vi "peak -- draw -- fit related.vi"() -> ()   [LabVIEW 2010]
uses:
  circle corners.ctl
  lorentzian.ctl
  wavepacket.ctl
  complex region.ctl
panel:
  in  "complex region 2":T1
  in  "parameters: wavepacket  2":T2={"R"=0.5, "wave number"=22.0, "delta k"=7.0, "radii vector"=[], "radial section"=[], "wave vector"=22.0, "wavepacket is"=TRUE} {"delta k" format="%#_3f"; "wave number" format="%#_3f"; "R" format="%#_3f"}
  in  "lorentzian":T3={"Amplitude"=-1.0311345636926572, "omega(0)"=-1.0311345636926572, "Gamma"=-1.0311345636926572, "phase"=-1.0311345636926572, "Q"=-1.0311345636926572, "Norm  Ampl"=-1.0311345636926572, "z (inf)"=-1.0311345636926572+0.0i, "4corners"={"z (-pi/2)"=-1.0311345636926572+0.5736824521422934i, "z(inf)"=-0.5200164984937075+1.0975277942502903i, "z (pi/2)"=-1.0311345636926572+0.5736824521422934i, "z center"=-0.5136528600391839+0.580046090596817i, "z(0)"=-0.5200164984937075+1.0975277942502903i, "radius"=-1.0311345636926572}} {"z (inf)" format="%#9_9f"; "Q" format="%#9_9f"; "phase" format="%#9_9f"; "Gamma" format="%#9_9f"; "omega(0)" format="%#9_9f"}
  out "Plot: complex plane":cluster{dbl[], dbl[]}[](graph)=[{array[1389 elements], array[1389 elements]}, {[0.4353850246464146, 0.43182331903139287, 0.4211943724115363, 0.403665809624465, 0.379514066576387, 0.3491200306827224, 0.3129630340460312, 0.27161329410241697, 0.22572292095192775, 0.176015633192727, 0.12327534444647162, 0.06833380057221139, 0.012057462537330959, -0.04466615818950484, -0.10094249622438536, -0.1558840400986455, -0.20862432884490087, -0.25833161660410175, -0.3042219897545908, -0.3455717296982051, -0.3817287263348962, -0.4121227622285608, -0.43627450527663886, -0.4538030680637101, -0.4644320146835667, -0.46799372029858843, -0.4644320146835667, -0.4538030680637101, -0.4362745052766388, -0.41212276222856076, -0.38172872633489613, -0.34557172969820504, -0.30422198975459075, -0.25833161660410153, -0.20862432884490062, -0.1558840400986455, -0.10094249622438527, -0.04466615818950476, 0.012057462537331146, 0.06833380057221167, 0.12327534444647154, 0.17601563319272698, 0.22572292095192786, 0.2716132941024171, 0.3129630340460314, 0.3491200306827225, 0.379514066576387, 0.403665809624465, 0.42119437241153634, 0.43182331903139287], [0.016304347826086918, 0.07291603744469696, 0.1286349268998374, 0.18258229601994944, 0.2339073625674127, 0.28180069958266507, 0.32550700053088333, 0.36433699093723537, 0.39767829865710114, 0.4250051113506065, 0.44588646885732824, 0.4599930596954671, 0.4671024145006366, 0.4671024145006366, 0.45999305969546705, 0.44588646885732824, 0.4250051113506065, 0.3976782986571011, 0.36433699093723537, 0.3255070005308833, 0.2818006995826651, 0.23390736256741268, 0.18258229601994933, 0.1286349268998374, 0.07291603744469691, 0.016304347826086772, -0.04030734179252315, -0.09602623124766366, -0.14997360036777574, -0.2012986669152389, -0.24919200393049135, -0.2928983048787095, -0.3317282952850616, -0.36506960300492736, -0.39239641569843275, -0.4132777732051544, -0.4273843640432933, -0.4344937188484628, -0.4344937188484628, -0.4273843640432932, -0.41327777320515446, -0.39239641569843264, -0.36506960300492725, -0.3317282952850614, -0.2928983048787093, -0.249192003930491, -0.20129866691523887, -0.14997360036777554, -0.09602623124766342, -0.040307341792522926]}, {[-0.02920754195733423, -0.0279172225442095, -0.02662690313108477, -0.025336583717960035, -0.024046264304835304, -0.022755944891710574, -0.021465625478585843, -0.020175306065461113, -0.01888498665233638, -0.017594667239211652, -0.016304347826086918, -0.015014028412962187, -0.013723708999837457, -0.012433389586712727, -0.011143070173587993, -0.009852750760463262, -0.008562431347338532, -0.007272111934213801, -0.005981792521089071, -0.004691473107964337], [-0.4352006873460732, -0.3900501838288572, -0.3448996803116412, -0.29974917679442514, -0.25459867327720914, -0.20944816975999314, -0.16429766624277709, -0.11914716272556108, -0.07399665920834508, -0.028846155691129083, 0.016304347826086918, 0.061454851343302974, 0.10660535486051903, 0.15175585837773498, 0.19690636189495103, 0.24205686541216698, 0.28720736892938303, 0.3323578724465991, 0.37750837596381503, 0.4226588794810311]}, {[-0.46780938299824704, -0.42265887948103104, -0.37750837596381503, -0.332357872446599, -0.287207368929383, -0.24205686541216698, -0.19690636189495092, -0.15175585837773492, -0.10660535486051892, -0.06145485134330292, -0.016304347826086918, 0.02884615569112914, 0.0739966592083452, 0.11914716272556114, 0.1642976662427772, 0.20944816975999314, 0.2545986732772092, 0.29974917679442525, 0.3448996803116412, 0.39005018382885726], [0.02920754195733423, 0.0279172225442095, 0.02662690313108477, 0.025336583717960035, 0.024046264304835304, 0.022755944891710574, 0.021465625478585843, 0.020175306065461113, 0.01888498665233638, 0.017594667239211652, 0.016304347826086918, 0.015014028412962187, 0.013723708999837457, 0.012433389586712727, 0.011143070173587993, 0.009852750760463262, 0.008562431347338532, 0.007272111934213801, 0.005981792521089071, 0.004691473107964337]}, {[0.01005665579823264, 0.007744432577840361, 0.005417179652517198, 0.003076351479586171, 0.0007234110004580747, -0.0016401712736591172, -0.00401291818078202, -0.006393346831329957, -0.008779969534882585, -0.011171294729938152, -0.013565827916090699, -0.015962072588044322, -0.018358531170880203, -0.02075370595599212, -0.023146100037105728, -0.025534218245796075, -0.027916568085919358, -0.030291660666374353, -0.032658011631610834, -0.03501414208930362], [0.10847338189925305, 0.10910353702052725, 0.10967569566929894, 0.11018950026503718, 0.11064462969659473, 0.11104079952289196, 0.11137776215068329, 0.11165530698929499, 0.11187326058223739, 0.1120314867156096, 0.11212988650322873, 0.11216839844843059, 0.11214699848250304, 0.11206569997972819, 0.11192455374902387, 0.1117236480021898, 0.11146310829877795, 0.11114309746762203, 0.11076381550507473, 0.11032549945001648]}, {[0.014540048997765252, 0.011834570421475052, 0.00911150593724143, 0.006372557371727504, 0.003619436478630049, 0.0008538638688893457, -0.0019224320646368132, -0.0047077162273623414, -0.007500247907350391, -0.010298281863201853, -0.013100069414774205, -0.015903859536049864, -0.018707899949470363, -0.021510438221052725, -0.024309722855603812, -0.027104004391347636, -0.029891536493282165, -0.0326705770445818, -0.03543938923536362, -0.038196242648137146], [0.12414918948458693, 0.12488651932597554, 0.125555988844679, 0.12615717964404025, 0.12668971599937934, 0.12715326509280894, 0.12754753722123485, 0.12787228597741096, 0.1281273084039356, 0.12831244512009365, 0.12842758042146385, 0.12847264235223071, 0.12844760275015438, 0.128352477264171, 0.1281873253446129, 0.12795225020605383, 0.1276473987628034, 0.12727296153709028, 0.1268291725399921, 0.1263163091251861]}]
  out "Plot: linear map":cluster{dbl[], dbl[]}[](graph)
  out "Plot: geometry":cluster{dbl, dbl}[](graph)
  out "Plot: phase around center":cluster{dbl[], dbl[]}[](graph)=[{array[1389 elements], array[1389 elements]}, {[3015.8552146531347, 3016.2383756063605, 3016.6215365595863], [1.7830935388456814, 3.353889865640578, 4.924686192435475]}, {array[1389 elements], array[1389 elements]}]
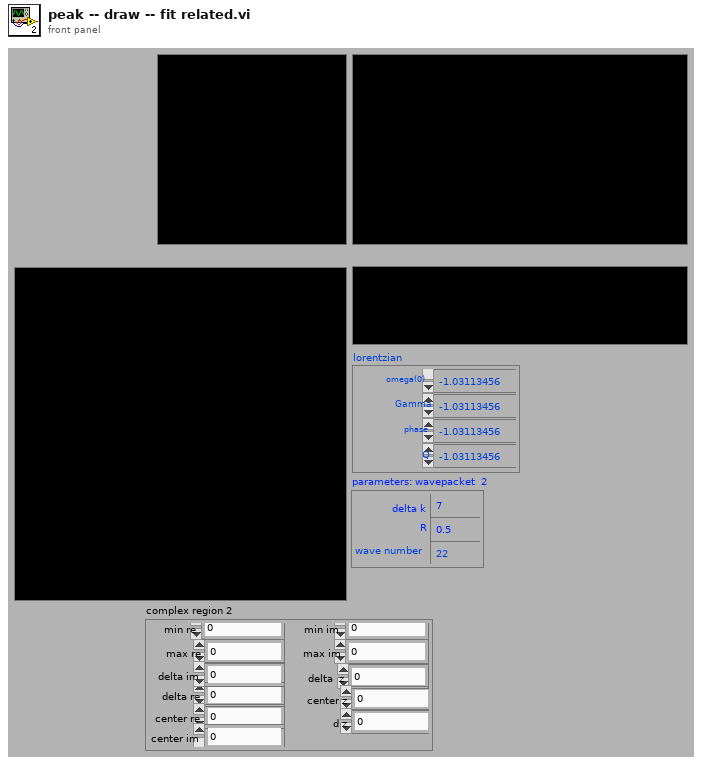
[diagram p1: front panel]
types:
  T1 = typedef "complex region.ctl" = cluster{"max re":dbl, "min re":dbl, "max im":dbl, "min im":dbl, "delta re":dbl, "delta im":dbl, "center re":dbl, "delta  z":cdb, "center im":dbl, "center z":cdb, "d im":dbl, "d re":dbl, "d z":cdb}
  T2 = typedef "wavepacket.ctl" = cluster{"R":dbl, "wave number":dbl, "delta k":dbl, "radii vector":dbl[], "radial section":cdb[], "wave vector":dbl, "wavepacket is":bool}
  T3 = typedef "lorentzian.ctl" = cluster{"Amplitude":dbl, "omega(0)":dbl, "Gamma":dbl, "phase":dbl, "Q":dbl, "Norm  Ampl":dbl, "z (inf)":cdb, "4corners":T4}
  T4 = typedef "circle corners.ctl" = cluster{"z (-pi/2)":cdb, "z(inf)":cdb, "z (pi/2)":cdb, "z center":cdb, "z(0)":cdb, "radius":dbl}
  T5 = typedef "single fit parameters.ctl" = cluster{"number of 2D grid points":i32, "# of points in pond":i32, "# of points in window":i32, "decimation threshold":i32, "normalization factor":dbl, "pond scale factor ":dbl, "normalized z":cdb[], "decimated z":cdb[], "decimated omega":dbl[], "omega in window":dbl[], "z in window":cdb[], "data center":cdb, "inverse":cdb[], "linear ":cdb[], "omega around":dbl[], "phase around center":dbl[], "fit for phase around senter ":dbl[], "three points":cluster{dbl[], dbl[]}, "max omega":dbl, "min omega":dbl}
  T6 = typedef "omega map parameters.ctl" = cluster{"map method":enum16{"simple", "less trivial", "around center", "geometry"}, "2:window factor":i32, "left":dbl, "right":dbl, "omega":dbl, "gamma":dbl, "theta0":dbl, "use points":enum16{"all in window", "decimated"}, "z(inf) method":enum16{"median", "method 2", "histogram"}}
  T7 = cluster{"omega in window":void, "phase around center":void}
  T8 = cluster{"omega in window":void, "f(X,a)":dbl[]}[]
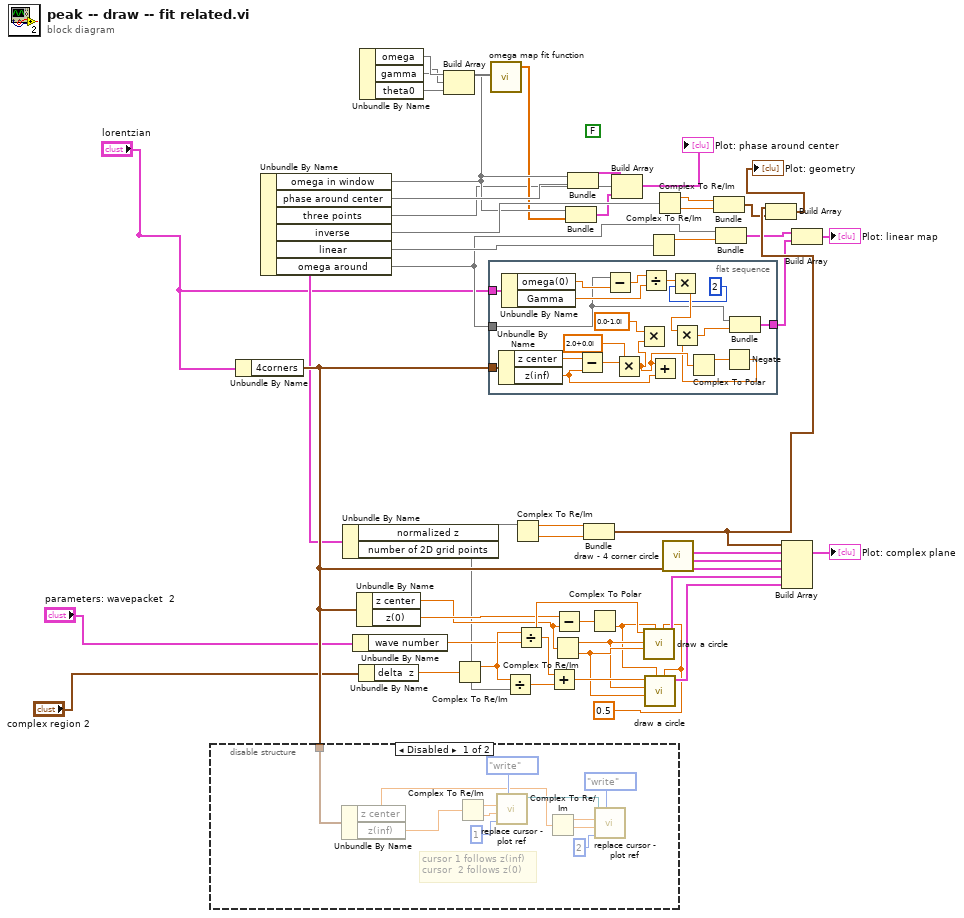
[diagram p0: block diagram]
diagram:
  w14 = 0.5
  (unwired) FALSE
  n1 = Unbundle By Name("lorentzian") -> ("4corners"=w50:T4)
  n2 = disable-structure shown="Disabled" {
    disable-tunnel: w50 -> [w65 _]
    frame Disabled {
      # "cursor 1 follows z(inf)\ncursor  2 follows z(0)"
      n3 = Unbundle By Name(w65) -> ("z center"=w53:cdb, "z(inf)"=w54:cdb)
      n4 = Complex To Re/Im(x + iy=w54) -> (x=w61:dbl, y=w60:dbl)
      n5 = call "replace cursor - plot ref.vi"("action"=enum16{"", "read", "write"}."write" ("Enum"), "cursor index"=1, "new  Y"=w60, "new X"=w61) -> ("Plot ref out"=w55:refnum<vi>, "Plot ref in"=w64:refnum<vi>)  [unwired: 4 in, 2 out]
      n6 = Complex To Re/Im(x + iy=w53) -> (x=w57:dbl, y=w56:dbl)
      n7 = call "replace cursor - plot ref.vi"("action"=enum16{"", "read", "write"}."write" ("Enum"), "cursor index"=2, "new  Y"=w56, "new X"=w57, "Plot ref in"=w55) -> ()  [unwired: 4 in, 3 out]
    }
    frame Enabled {
    }
  }
  n8 = Unbundle By Name() -> (w49:T5, "omega in window"=w30, "phase around center"=w37, "three points"=w28, "inverse"=w41, "linear"=w40, "omega around"=w39)
  n9 = Unbundle By Name(w49) -> ("normalized z"=w9, "number of 2D grid points"=w4)
  n10 = Unbundle By Name("parameters: wavepacket  2") -> ("wave number"=w10:dbl)
  n11 = Unbundle By Name(w50) -> ("z center"=w5:cdb, "z(0)"=w17:cdb)
  n12 = Unbundle By Name("complex region 2") -> ("delta  z"=w11:cdb)
  n13 = Unbundle By Name() -> (w51:T6, "omega"=w34, "gamma"=w33, "theta0"=w32)
  n14 = Build Array(w34, w33, w32) -> (w31:void[])
  n15 = Complex To Re/Im(x + iy=w11) -> (x=w12:dbl)  [unwired: 1 out]
  n16 = flat-sequence {
    tunnel: "lorentzian" -> [w84]
    tunnel: w50 -> [w83]
    tunnel: w39 -> [w72]
    tunnel: [w71] -> w38
    frame #0 {
      n17 = Unbundle By Name(w83) -> ("z center"=w82:cdb, "z(inf)"=w80:cdb)
      n18 = Unbundle By Name(w84) -> ("omega(0)"=w78:dbl, "Gamma"=w76:dbl)
      n19 = Subtract(x=w82, y=w80) -> (x-y=w81:cdb)
      n20 = Subtract(x=w72, y=w78) -> (x-y=w77:dbl)
      n21 = Multiply(x=w81, y=cdb 2.0+0.0i) -> (x*y=w68:cdb)
      n22 = Multiply(x=cdb 0.0-1.0i ("y"), y=w68) -> ()  [unwired: 1 out]
      n23 = Divide(x=w77, y=w76) -> (x/y=w75:dbl)
      n24 = Add(x=w68, y=w80) -> ()  [unwired: 1 out]
      n25 = Multiply(x=w75, y=2) -> (x*y=w73:dbl)
      n26 = Complex To Polar(r * e^(i*theta)=w68) -> (r=w67:dbl)  [unwired: 1 out]
      n27 = Negate(x=w67) -> (-x=w66:dbl)
      n28 = Multiply(x=w73, y=w66) -> (x*y=w69:dbl)
      n29 = Bundle("omega around"=w72, w69) -> (w71:cluster{"omega around":void, dbl})  [unwired: 1 in]
    }
  }
  n30 = call "omega map fit function.vi"("X"=w30, "a"=w31) -> ("f(X,a)"=w29:dbl[])  [unwired: 2 in, 2 out]
  n31 = Divide(x=w12, y=w4) -> (x/y=w13:dbl)
  n32 = Complex To Re/Im(x + iy=w9) -> (x=w26:dbl, y=w25:dbl)
  n33 = Divide(x=w12, y=w10) -> (x/y=w22:dbl)
  n34 = Add(x=w22, y=w13) -> (x+y=w21:dbl)
  n35 = Complex To Re/Im(x + iy=w5) -> (x=w18:dbl, y=w19:dbl)
  n36 = Subtract(x=w17, y=w5) -> (x-y=w16:cdb)
  n37 = Bundle("omega in window"=w30, "f(X,a)"=w29) -> (w27:cluster{"omega in window":void, "f(X,a)":dbl[]})  [unwired: 1 in]
  n38 = Bundle("omega in window"=w30, "phase around center"=w37) -> (w36:T7)  [unwired: 1 in]
  n39 = Bundle(w26, w25) -> (w52:cluster{dbl, dbl})  [unwired: 1 in]
  n40 = Complex To Polar(r * e^(i*theta)=w16) -> (theta=w15:dbl)  [unwired: 1 out]
  n41 = Build Array(w36, w28, w27) -> (→"Plot: phase around center":T8)
  n42 = call "draw a circle.vi"("angular arc bounds"=w14, "angular arc center"=w15, "center Y"=w19, "center x"=w18, "radius"=w22) -> ("output cluster"=w23:cluster{dbl[], dbl[]})  [unwired: 6 in]
  n43 = call "draw a circle.vi"("angular arc bounds"=w14, "angular arc center"=w15, "center Y"=w19, "center x"=w18, "radius"=w21) -> ("output cluster"=w20:cluster{dbl[], dbl[]})  [unwired: 6 in]
  n44 = Complex To Re/Im(x + iy=w40) -> (x=w44:dbl)  [unwired: 1 out]
  n45 = Complex To Re/Im(x + iy=w41) -> (x=w47:dbl, y=w46:dbl)
  n46 = call "draw - 4 corner circle.vi"("4corners"=w50) -> ("line two"=w6:cluster{dbl[], dbl[]}, "line one"=w7:cluster{dbl[], dbl[]}, "circle"=w8:cluster{dbl[], dbl[]})  [unwired: 8 in]
  n47 = Bundle(w47, w46) -> (w45:cluster{dbl, dbl})  [unwired: 1 in]
  n48 = Bundle("omega around"=w39, w44) -> (w43:cluster{"omega around":void, dbl})  [unwired: 1 in]
  n49 = Build Array(w52, w45) -> (→"Plot: geometry":cluster{dbl, dbl}[])
  n50 = Build Array(w52, w8, w7, w6, w23, w20) -> (→"Plot: complex plane":cluster{dbl[], dbl[]}[])
  n51 = Build Array(w43, w38) -> (→"Plot: linear map":cluster{"omega around":void, dbl}[])
